vi "Enqueue.vi"(8 "error in (no error)":errorcluster, 9 "Data":variant, 10 "State":string, 11 "Master in":refnum<class "Master.lvclass">) -> (0 "error out":errorcluster, 3 "Master out":refnum<class "Master.lvclass">)   [LabVIEW 2014, in "Master.lvclass"]
uses:
  Master.lvclass
  Master.lvclass/Master.ctl
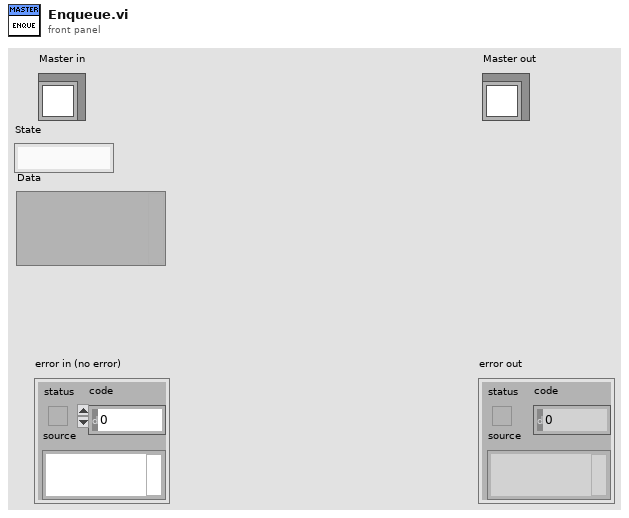
[diagram p1: front panel]
types:
  T1 = typedef "Control Library.lvlib/StateDatas.ctl" = cluster{"State":string, "Data":variant}
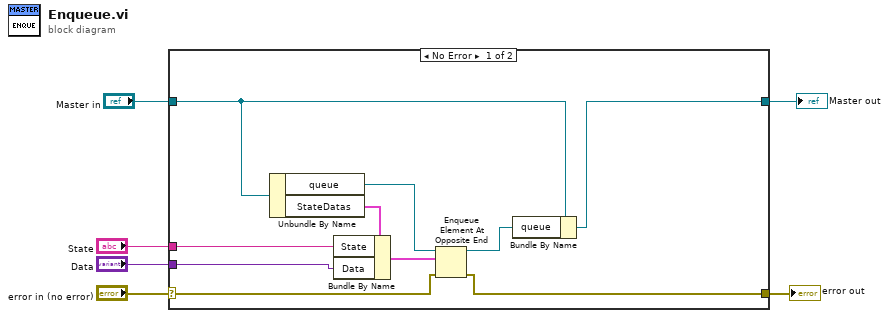
[diagram p0: block diagram]
diagram:
  n1 = case shown="No Error" "error in (no error)" {
    selector: "error in (no error)" -> [w12 w18]
    tunnel: [w11 w18] -> w5
    tunnel: [w13 w17] -> w3
    tunnel: "Master in" -> [w15 w17]
    tunnel: "State" -> [w8 _]
    tunnel: "Data" -> [w7 _]
    frame No Error {
      n2 = Unbundle By Name(w15) -> ("queue"=w16:refnum<queue>, "StateDatas"=w10:T1)
      n3 = Bundle By Name(cluster=w10, "State"=w8, "Data"=w7) -> (w9:T1)
      n4 = Enqueue Element At Opposite End(queue=w16, element=w9, error in (no error)=w12) -> (queue out=w14:refnum<queue>, error out=w11:errorcluster)  [unwired: 1 in, 1 out]
      n5 = Bundle By Name(cluster=w15, "queue"=w14) -> (w13:refnum<class "Master.lvclass">)
    }
    frame Error {
    }
  }
  "error out" <- w5
  "Master out" <- w3
